vi "Write sequence info to MAT file.vi"(4 "Header2 file data":T1, 6 "Number of frames":u32, 7 "first frame number":u32, 8 "error in":errorcluster, 9 "Header file data":T2 {"Pixel depth" items=["8 bits", "16 bits", "Float", "Complex", "RGB", "HSL"]; "time of 1st frame, \nsec since 1/1/04" format="%.2f"}, 10 "Movie file name":string, 11 "Description Info":string) -> (0 "error out":errorcluster)   [LabVIEW 2016]
doc: "Writes a documentation file (in Matlabs MAT format) to accompany an AVI or stacked-TIFF movie. The only contents of the file will be a structure named 'vid'. Read the file using the Matlab 'load' command:\n\n>> load 16.01.mat\n>> vid\n\nvid = \n\n moviefile: '\\\\Jg_i\\c-drive\\LabView development\\Glimpse\\junk4\\16.01.tif'\n username: 'gelles'\n description: 'GLIMPSE v. 36 (8/04)'\n nframes: 5\n time1: 3.1555e+009\n ttb: [300 334 367 400 434]\n depth: 0\n width: 32\n height: 32\n\nNotes on the elements of the structure:\n\nnframes -- number of frames in the movie\ntime1 -- time of acquisition of the first frame in seconds from Jan 1, 1904\nttb -- timestamps of frames in milliseconds\ndepth -- 0 <-> 8-bit; 1 <-> 16-bit\nwidth, height -- image width and height in pixels\n\n2/10/06 -- added offset array infomation to mat output"
uses:
  Header file data.ctl
  Seq file v 1/Offset table.ctl
  Seq file v 1/Offset.ctl
  Seq file v 1/file number.ctl
  Header2 file data.ctl
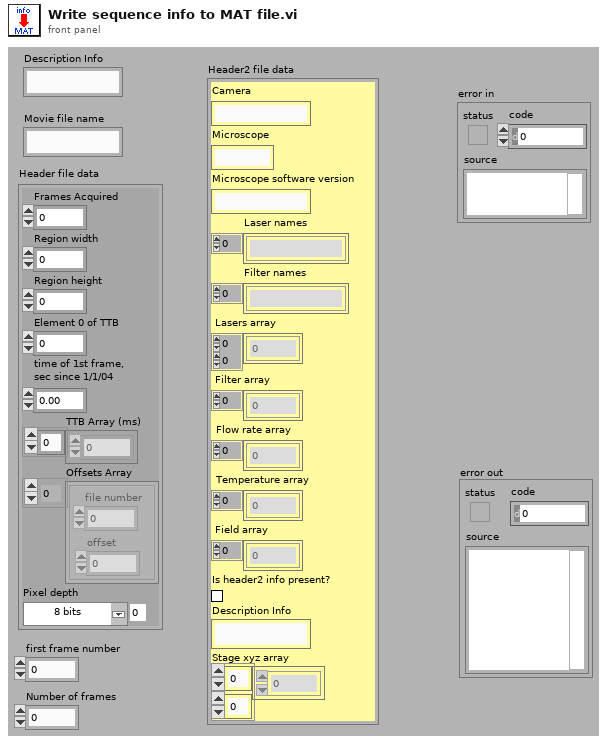
[diagram p1: front panel]
types:
  T1 = typedef "Header2 file data.ctl" = cluster{"Camera":string, "Microscope":string, "Microscope software version":string, "Laser names":string[], "Filter names":string[], "Lasers array":u16[][], "Filter array":u16[], "Flow rate array":dbl[], "Temperature array":dbl[], "Field array":u16[], "Is header2 info present?":bool, "Description Info":string, "Stage xyz array":dbl[][]}
  T2 = typedef "Header file data.ctl" = cluster{"Frames Acquired":u32, "Region width":i32, "Region height":i32, "Element 0 of TTB":u32, "time of 1st frame, \nsec since 1/1/04":dbl, "TTB Array (ms)":u32[], "Offsets Array":T3, "Pixel depth":u32}
  T3 = typedef "Offset table.ctl" = cluster{"offset":T4, "file number":T5}[]
  T4 = typedef "Offset.ctl" = i32
  T5 = typedef "file number.ctl" = u8
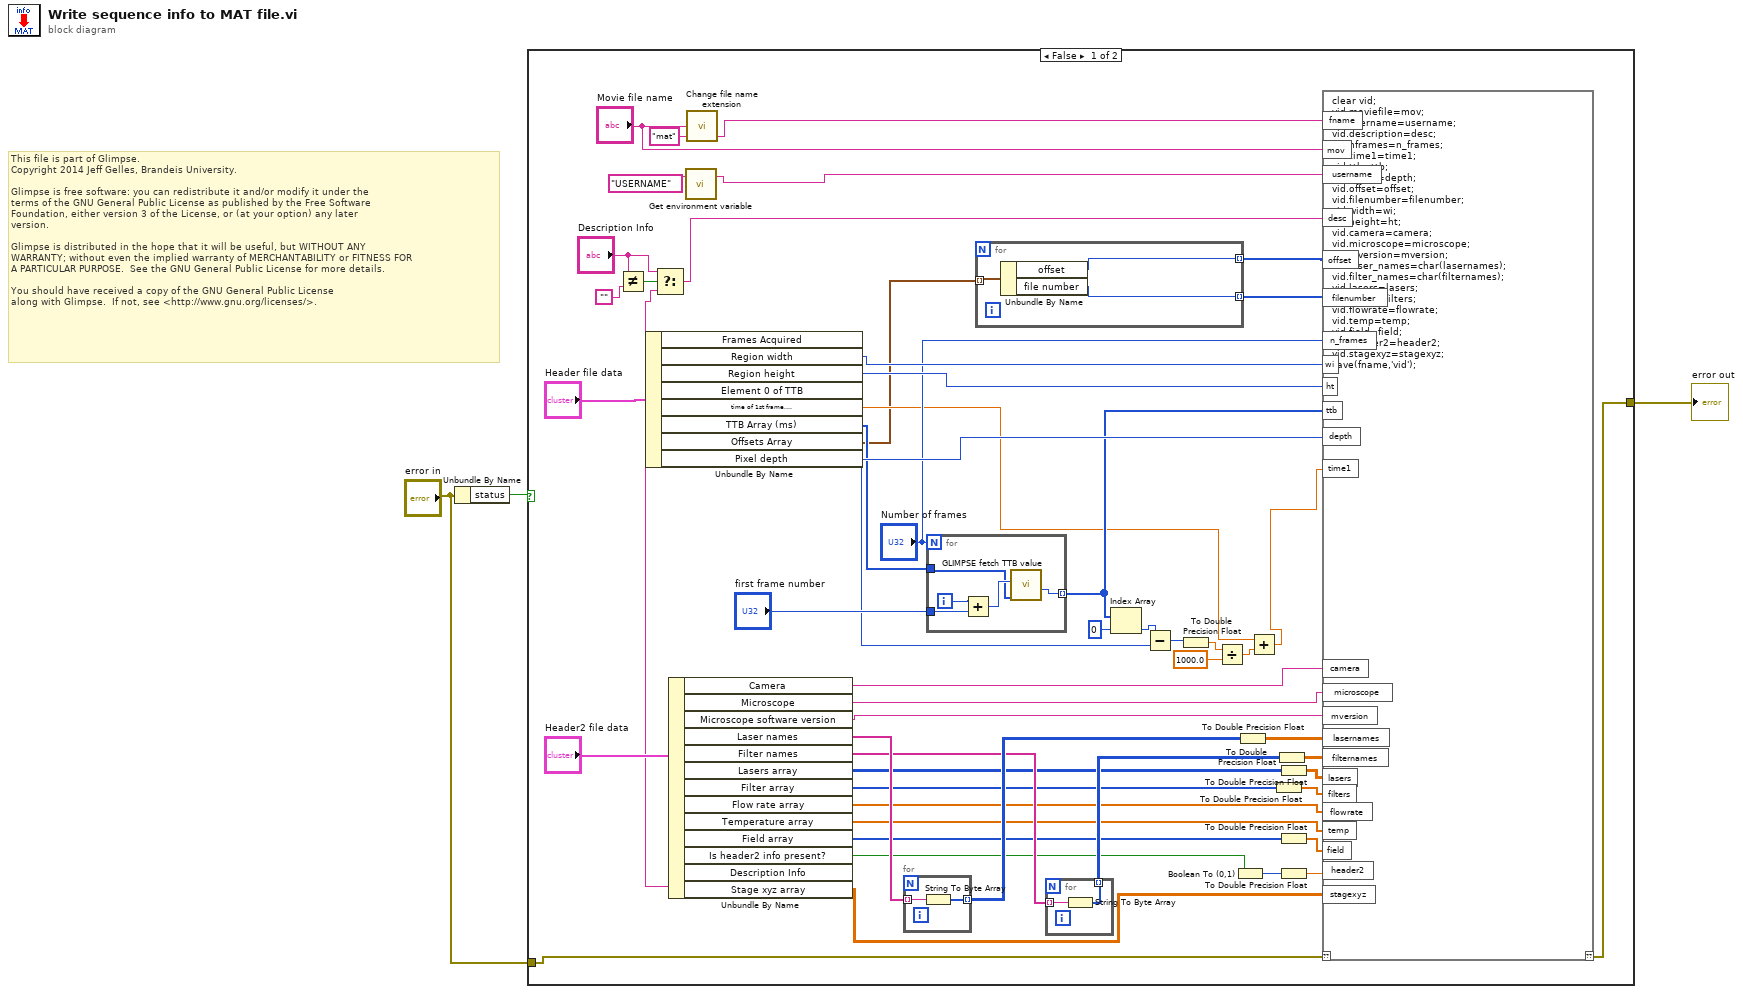
[diagram p0: block diagram]
diagram:
  # "This file is part of Glimpse. \nCopyright 2014 Jeff Gelles, Brandeis University.    \n\nGlimpse is free software: you can redistribute it and/or modify it under the \nterms of the GNU General Public License as published by the Free Software \nFoundation, either version 3 of the License, or (at your option) any later \nversion.\n\nGlimpse is distributed in the hope that it will be useful, but WITHOUT ANY \nWARRANTY; without even the implied warranty of MERCHANTABILITY or FITNESS FOR \nA PARTICULAR PURPOSE.  See the GNU General Public License for more details.\n\nYou should have received a copy of the GNU General Public License\nalong with Glimpse.  If not, see <http://www.gnu.org/licenses/>."
  n1 = Unbundle By Name("error in") -> ("status"=w3:bool)
  n2 = case shown="False" w3 {
    tunnel: "error in" -> [w49 w70]
    tunnel: [w47 w70] -> w1
    frame False {
      n3 = Not Equal?(x="Description Info", y="") -> (x != y?=w14:bool)
      n4 = Unbundle By Name("Header file data") -> ("Region width"=w50:i32, "Region height"=w51:i32, "Element 0 of TTB"=w40:u32, "time of 1st frame, \nsec since 1/1/04"=w35:dbl, "TTB Array (ms)"=w45:u32[], "Offsets Array"=w33:T3, "Pixel depth"=w52:u32)  [unwired: 1 out]
      n5 = Unbundle By Name("Header2 file data") -> ("Camera"=w29:string, "Microscope"=w28:string, "Microscope software version"=w27:string, "Laser names"=w26:string[], "Filter names"=w24:string[], "Lasers array"=w22:u16[][], "Filter array"=w21:u16[], "Flow rate array"=w20:dbl[], "Temperature array"=w19:dbl[], "Field array"=w18:u16[], "Is header2 info present?"=w16:bool, "Description Info"=w12:string, "Stage xyz array"=w10:dbl[][])
      n6 = Select(t="Description Info", s=w14, f=w12) -> (s? t:f=w11:string)
      n7 = call "Get environment variable.vi"("Variable name"="USERNAME") -> ("Value"=w53:string)  [unwired: 2 out]
      n8 = call "Change file name extension.vi"("New Extension (no period)"="mat", "Path String In"="Movie file name") -> ("New Path String Out"=w54:string)  [unwired: 3 out]
      n9 = for {
        tunnel: w26 -> [w59] mode=indexing
        tunnel: [w58] -> w25 mode=indexing
        n10 = String To Byte Array(string=w59) -> (unsigned byte array=w58:u8[])
      }
      n11 = for {
        N: "Number of frames" -> [_]
        tunnel: w45 -> [w66]
        tunnel: "first frame number" -> [w68]
        tunnel: [w65] -> w43 mode=indexing
        i -> [w69]
        n12 = Add(x=w69, y=w68) -> (x+y=w67:u32)
        n13 = call "GLIMPSE fetch TTB value.vi"("Array of TTB Values (ms)"=w66, "Logical Frame Number\n(starting with zero)"=w67) -> ("TTB value out"=w65:u32)  [unwired: 6 out]
      }
      n14 = for {
        tunnel: w33 -> [w64] mode=indexing
        tunnel: [w63] -> w32 mode=indexing
        tunnel: [w62] -> w31 mode=indexing
        n15 = Unbundle By Name(w64) -> ("offset"=w63:T4, "file number"=w62:T5)
      }
      n16 = for {
        tunnel: w24 -> [w61] mode=indexing
        tunnel: [w60] -> w23 mode=indexing
        n17 = String To Byte Array(string=w61) -> (unsigned byte array=w60:u8[])
      }
      n18 = Index Array(array=w43, index=0) -> (element=w41:u32)
      n19 = Subtract(x=w41, y=w40) -> (x-y=w39:u32)
      n20 = To Double Precision Float(number=w39) -> (double precision float=w38:dbl)
      n21 = Divide(x=w38, y=1000.0) -> (x/y=w36:dbl)
      n22 = Boolean To (0,1)(Boolean=w16) -> (0, 1=w17:i16)
      n23 = To Double Precision Float(number=w25) -> (double precision float=w9:dbl[][])
      n24 = Add(x=w35, y=w36) -> (x+y=w34:dbl)
      n25 = To Double Precision Float(number=w21) -> (double precision float=w6:dbl[])
      n26 = To Double Precision Float(number=w23) -> (double precision float=w4:dbl[][])
      n27 = To Double Precision Float(number=w22) -> (double precision float=w5:dbl[][])
      n28 = To Double Precision Float(number=w18) -> (double precision float=w7:dbl[])
      n29 = To Double Precision Float(number=w17) -> (double precision float=w8:dbl)
      n30 = script code="clear vid;\nvid.moviefile=mov;\nvid.username=username;\nvid.description=desc;\nvid.nframes=n_frames;\nvid.time1=time1;\nvid.ttb=ttb;\nvid.depth=depth;\nvid.offset=offset;\nvid.filenumber=filenumber;\nvid.width=wi;\nvid.height=ht;\nvid.camera=camera;\nvid.microscope=microscope;\nvid.mversion=mversion;\nvid.laser_names=char(lasernames);\nvid.filter_names=char(filternames);\nvid.lasers=lasers;\nvid.filters=filters;\nvid.flowrate=flowrate;\nvid.temp=temp;\nvid.field=field;\nvid.header2=header2;\nvid.stagexyz=stagexyz;\nsave(fname,'vid');"("??"=w49, "fname"=w54, "username"=w53, "n_frames"="Number of frames", "wi"=w50, "ht"=w51, "ttb"=w43, "depth"=w52, "time1"=w34, "desc"=w11, "mov"="Movie file name", "offset"=w32, "filenumber"=w31, "camera"=w29, "microscope"=w28, "mversion"=w27, "lasernames"=w9, "filternames"=w4, "lasers"=w5, "filters"=w6, "flowrate"=w20, "temp"=w19, "field"=w7, "header2"=w8, "stagexyz"=w10) -> ("??"=w47:errorcluster)
    }
    frame True {
    }
  }
  "error out" <- w1
